vi "EXA_Load_State_File.vi"(8 "error in":errorcluster, 10 "Path":path, 11 "VISA resource name":refnum<visa-resource-name>) -> (0 "error out":errorcluster, 3 "VISA resource name":refnum<visa-resource-name>)   [LabVIEW 2016]
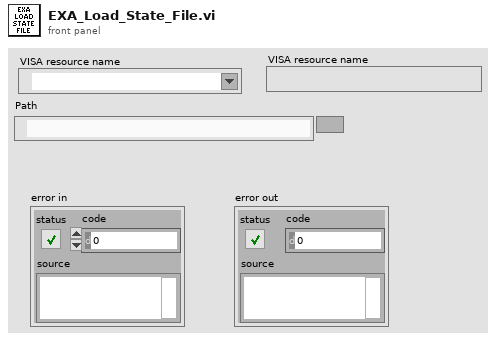
[diagram p1: front panel]
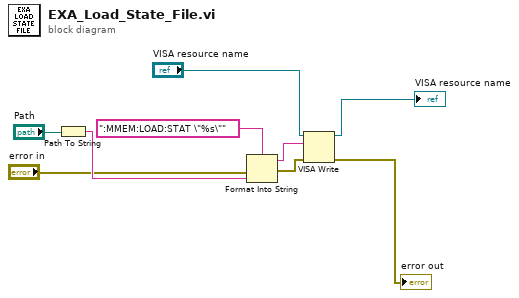
[diagram p0: block diagram]
diagram:
  n1 = Path To String(path="Path") -> (string=w2:string)
  n2 = Format Into String(format string=":MMEM:LOAD:STAT \"%s\"", error in="error in", w2) -> (resulting string=w4:string, error out=w7:errorcluster)  [unwired: 1 in]
  n3 = VISA Write(VISA resource name="VISA resource name", write buffer=w4, error in (no error)=w7) -> (VISA resource name out=→"VISA resource name":refnum<visa-resource-name>, error out=→"error out":errorcluster)  [unwired: 1 out]
